vi "readSingle.vi"(0 "refer":refnum<queue>, 1 "index":i32, 2 "wait":bool, 5 "errorIn":errorcluster) -> (11 "remark1":string, 13 "remark 2":string, 14 "refer":refnum<queue>, 15 "to":string, 16 "data":variant, 17 "vaildData":bool, 18 "from":string, 19 "errorOut":errorcluster)   [LabVIEW 2017]
uses:
  models/EMSGData.ctl
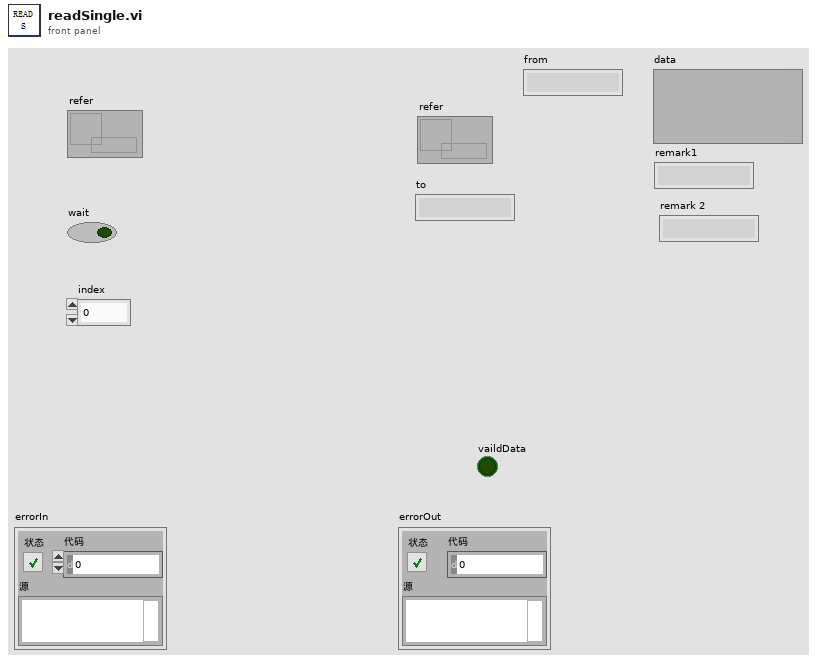
[diagram p1: front panel]
types:
  T1 = typedef "EMSGData.ctl" = cluster{"to":string, "from":string, "data":variant, "remark1":string, "remark 2":string}
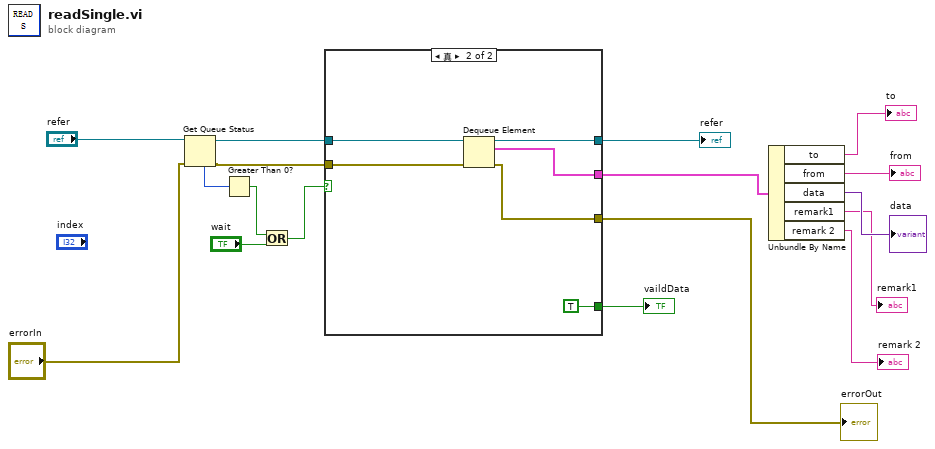
[diagram p0: block diagram]
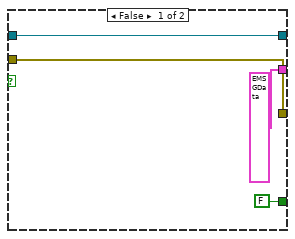
[diagram p2: hidden frame]
diagram:
  n1 = Get Queue Status(queue="refer", error in (no error)="errorIn") -> (queue out=w16:refnum<queue>, error out=w13:errorcluster, # elements in queue=w15:i32)  [unwired: 1 in, 5 out]
  n2 = Greater Than 0?(x=w15) -> (x > 0?=w11:bool)
  n3 = Or(x=w11, y="wait") -> (x .or. y?=w10:bool)
  n4 = case shown="真" w10 {
    tunnel: [w21 w27] -> w17
    tunnel: [T1 {"to"="", "from"="", "data"=variant, "remark1"="", "remark 2"=""} ("EMSGData") w26] -> w7
    tunnel: [w20 w25] -> w6
    tunnel: w16 -> [w21 w24]
    tunnel: w13 -> [w20 w23]
    tunnel: [FALSE TRUE] -> w9
    frame False {
    }
    frame True {
      n5 = Dequeue Element(queue=w24, error in (no error)=w23) -> (queue out=w27:refnum<queue>, element=w26:T1, error out=w25:errorcluster)  [unwired: 1 in, 1 out]
    }
  }
  "refer" <- w17
  "errorOut" <- w6
  "vaildData" <- w9
  n6 = Unbundle By Name(w7) -> ("to"=→"to":string, "from"=→"from":string, "data"=→"data":variant, "remark1"=→"remark1":string, "remark 2"=→"remark 2":string)
